vi "Check_SF.vi"(8 "error in (no error)":errorcluster, 11 "Limit":string) -> (0 "error out":errorcluster, 2 "TestResult":bool, 3 "TestData":string)   [LabVIEW 2013]
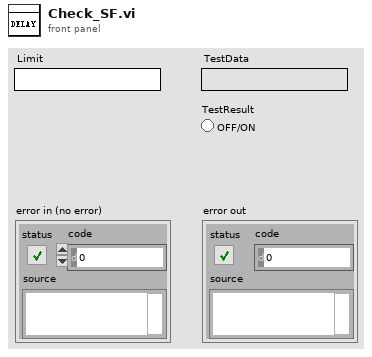
[diagram p1: front panel]
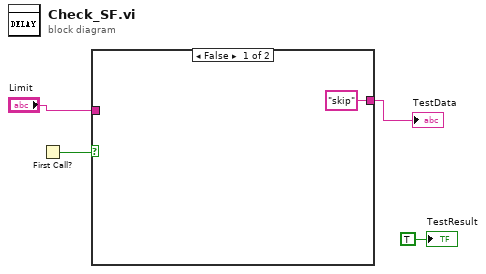
[diagram p0: block diagram]
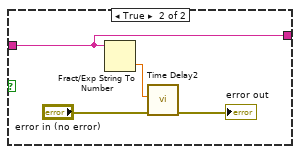
[diagram p2: hidden frame]
diagram:
  n1 = First Call?() -> (First Call?: T/F=w1:bool)
  n2 = case shown="False" w1 {
    tunnel: "Limit" -> [_ w6]
    tunnel: ["skip" ("Limit") w6] -> w2
    frame False {
    }
    frame True {
      n3 = Fract/Exp String To Number(string=w6) -> (number=w7:dbl)  [unwired: 3 in, 1 out]
      n4 = call "Time Delay2"("error in (no error)"="error in (no error)", "Delay Time (s)"=w7) -> ("error out"=→"error out":errorcluster)  [unwired: 9 in]
    }
  }
  "TestData" <- w2
  "TestResult" <- TRUE ("TestResult")
